vi "Func-엑셀 데이터를 그래프로 출력.vi"() -> ()   [LabVIEW 2015] (continued)
3.3\t3.3\t13.424\n3.3\t3.3\t13.421\n3.3\t3.3\t13.421\n3.3\t3.3\t13.424\n3.3\t3.3\t13.424\n3.3\t3.3\t13.418\n3.3\t3.3\t13.417\n3.3\t3.3\t13.415\n3.3\t3.3\t13.412\n3.3\t3.3\t13.407\n3.3\t3.3\t13.404\n3.3\t3.3\t13.403\n3.3\t3.3\t13.401\n3.3\t3.3\t13.399\n3.3\t3.3\t13.397\n3.3\t3.3\t13.395\n3.3\t3.3\t13.394\n3.3\t3.3\t13.395\n3.3\t3.3\t13.394\n3.3\t3.3\t13.395\n3.3\t3.3\t13.391\n3.3\t3.3\t13.389\n3.3\t3.3\t13.387\n3.3\t3.3\t13.384\n3.3\t3.3\t13.385\n3.3\t3.3\t13.382\n3.3\t3.3\t13.381\n3.3\t3.3\t13.379\n3.3\t3.3\t13.379\n3.3\t3.3\t13.379\n3.3\t3.3\t13.376\n3.3\t3.3\t13.374\n3.3\t3.3\t13.375\n3.3\t3.3\t13.378\n3.3\t3.3\t13.375\n3.3\t3.3\t13.371\n3.3\t3.3\t13.367\n3.3\t3.3\t13.366\n3.3\t3.3\t13.359\n3.3\t3.3\t13.358\n3.3\t3.3\t13.359\n3.3\t3.3\t13.357\n3.3\t3.3\t13.358\n3.3\t3.3\t13.356\n3.3\t3.3\t13.356\n3.3\t3.3\t13.352\n3.3\t3.3\t13.348\n3.3\t3.3\t13.343\n3.3\t3.3\t13.341\n3.3\t3.3\t13.34\n3.3\t3.3\t13.339\n3.3\t3.3\t13.336\n3.3\t3.3\t13.338\n3.3\t3.3\t13.337\n3.3\t3.3\t13.336\n3.3\t3.3\t13.335\n3.3\t3.3\t13.334\n3.3\t3.3\t13.335\n3.3\t3.3\t13.336\n3.3\t3.3\t13.334\n3.3\t3.3\t13.332\n3.3\t3.3\t13.331\n3.3\t3.3\t13.329\n3.3\t3.3\t13.327\n3.3\t3.3\t13.322\n3.3\t3.3\t13.321\n3.3\t3.3\t13.319\n3.3\t3.3\t13.317\n3.3\t3.3\t13.312\n3.3\t3.3\t13.309\n3.3\t3.3\t13.305\n3.3\t3.3\t13.302\n3.3\t3.3\t13.305\n3.3\t3.3\t13.308\n3.3\t3.3\t13.309\n3.3\t3.3\t13.31\n3.3\t3.3\t13.309\n3.3\t3.3\t13.304\n3.3\t3.3\t13.302\n3.3\t3.3\t13.299\n3.3\t3.3\t13.294\n3.3\t3.3\t13.29\n3.3\t3.3\t13.29\n3.3\t3.3\t13.289\n3.3\t3.3\t13.286\n3.3\t3.3\t13.284\n3.3\t3.3\t13.282\n3.3\t3.3\t13.282\n3.3\t3.3\t13.28\n3.3\t3.3\t13.276\n3.3\t3.3\t13.277\n3.3\t3.3\t13.277\n3.3\t3.3\t13.274\n3.3\t3.3\t13.273\n3.3\t3.3\t13.273\n3.3\t3.3\t13.277\n3.3\t3.3\t13.272\n3.3\t3.3\t13.268\n3.3\t3.3\t13.271\n3.3\t3.3\t13.269\n3.3\t3.3\t13.265\n3.3\t3.3\t13.258\n3.3\t3.3\t13.258\n3.3\t3.3\t13.257\n3.3\t3.3\t13.251\n3.3\t3.3\t13.249\n3.3\t3.3\t13.249\n3.3\t3.3\t13.25\n3.3\t3.3\t13.25\n3.3\t3.3\t13.246\n3.3\t3.3\t13.246\n3.3\t3.3\t13.241\n3.3\t3.3\t13.241\n3.3\t3.3\t13.24\n3.3\t3.3\t13.236\n3.3\t3.3\t13.234\n3.3\t3.3\t13.23\n3.3\t3.3\t13.232\n3.3\t3.3\t13.229\n3.3\t3.28\t13.225\n3.3\t3.28\t13.226\n3.3\t3.28\t13.227\n3.3\t3.28\t13.228\n3.3\t3.28\t13.229\n3.3\t3.28\t13.227\n3.3\t3.28\t13.229\n3.3\t3.28\t13.226\n3.3\t3.28\t13.222\n3.3\t3.28\t13.218\n3.3\t3.28\t13.214\n3.3\t3.28\t13.213\n3.3\t3.28\t13.211\n3.3\t3.28\t13.209\n3.3\t3.28\t13.212\n3.3\t3.28\t13.211\n3.3\t3.28\t13.21\n3.3\t3.28\t13.209\n3.3\t3.28\t13.209\n3.3\t3.28\t13.205\n3.3\t3.28\t13.202\n3.3\t3.28\t13.199\n3.3\t3.28\t13.199\n3.3\t3.28\t13.196\n3.3\t3.28\t13.194\n3.3\t3.28\t13.199\n3.3\t3.28\t13.2\n3.3\t3.28\t13.2\n3.3\t3.28\t13.193\n3.3\t3.28\t13.188\n3.3\t3.28\t13.185\n3.3\t3.28\t13.181\n3.3\t3.28\t13.18\n3.3\t3.28\t13.179\n3.3\t3.28\t13.181\n3.3\t3.28\t13.181\n3.3\t3.28\t13.181\n3.3\t3.28\t13.179\n3.3\t3.28\t13.178\n3.3\t3.28\t13.176\n3.3\t3.28\t13.179\n3.3\t3.28\t13.179\n3.3\t3.28\t13.176\n3.3\t3.28\t13.176\n3.3\t3.28\t13.171\n3.3\t3.28\t13.171\n3.3\t3.28\t13.167\n3.3\t3.28\t13.167\n3.3\t3.28\t13.166\n3.3\t3.28\t13.163\n3.3\t3.28\t13.165\n3.3\t3.28\t13.161\n3.3\t3.28\t13.16\n3.3\t3.28\t13.161\n3.3\t3.28\t13.16\n3.3\t3.3\t13.161\n3.3\t3.3\t13.157\n3.3\t3.3\t13.155\n3.3\t3.3\t13.154\n3.3\t3.3\t13.151\n3.3\t3.3\t13.151\n3.3\t3.3\t13.149\n3.3\t3.3\t13.15\n3.3\t3.3\t13.148\n3.3\t3.3\t13.148\n3.3\t3.3\t13.148\n3.3\t3.3\t13.145\n3.3\t3.3\t13.144\n3.3\t3.3\t13.143\n3.3\t3.3\t13.138\n3.3\t3.3\t13.135\n3.3\t3.3\t13.13\n3.3\t3.3\t13.128\n3.3\t3.3\t13.126\n3.3\t3.3\t13.124\n3.3\t3.3\t13.126\n3.3\t3.3\t13.128\n3.3\t3.3\t13.127\n3.3\t3.3\t13.125\n3.3\t3.3\t13.126\n3.3\t3.3\t13.126\n3.3\t3.3\t13.124\n3.3\t3.3\t13.121\n3.3\t3.3\t13.122\n3.3\t3.3\t13.119\n3.3\t3.3\t13.118\n3.3\t3.3\t13.114\n3.3\t3.3\t13.113\n3.3\t3.3\t13.111\n3.3\t3.3\t13.11\n3.3\t3.3\t13.108\n3.3\t3.3\t13.103\n3.3\t3.3\t13.101\n3.3\t3.3\t13.101\n3.3\t3.3\t13.097\n3.3\t3.3\t13.091\n3.3\t3.3\t13.091\n3.3\t3.3\t13.092\n3.3\t3.3\t13.094\n3.3\t3.3\t13.092\n3.3\t3.3\t13.09\n3.3\t3.3\t13.093\n3.3\t3.3\t13.091\n3.3\t3.3\t13.088\n3.3\t3.3\t13.083\n3.3\t3.3\t13.082\n3.3\t3.3\t13.082\n3.3\t3.3\t13.076\n3.3\t3.3\t13.076\n3.3\t3.3\t13.075\n3.3\t3.3\t13.077\n3.3\t3.3\t13.079\n3.3\t3.3\t13.079\n3.3\t3.3\t13.083\n3.3\t3.3\t13.082\n3.3\t3.3\t13.082\n3.3\t3.3\t13.082\n3.3\t3.3\t13.076\n3.3\t3.3\t13.075\n3.3\t3.3\t13.072\n3.3\t3.3\t13.07\n3.3\t3.3\t13.068\n3.3\t3.3\t13.062\n3.3\t3.3\t13.061\n3.3\t3.3\t13.06\n3.3\t3.3\t13.061\n3.3\t3.3\t13.061\n3.3\t3.3\t13.065\n3.3\t3.3\t13.066\n3.3\t3.3\t13.068\n3.3\t3.3\t13.064\n3.3\t3.3\t13.059\n3.3\t3.3\t13.057\n3.3\t3.3\t13.053\n3.3\t3.3\t13.051\n3.3\t3.3\t13.046\n3.3\t3.3\t13.05\n3.3\t3.3\t13.052\n3.3\t3.3\t13.05\n3.3\t3.3\t13.047\n3.3\t3.3\t13.044\n3.3\t3.3\t13.046\n3.3\t3.3\t13.046\n3.3\t3.3\t13.041\n3.3\t3.3\t13.04\n3.3\t3.3\t13.042\n3.3\t3.3\t13.044\n3.3\t3.3\t13.043\n3.3\t3.3\t13.039\n3.3\t3.3\t13.037\n3.3\t3.3\t13.037\n3.3\t3.3\t13.033\n3.3\t3.3\t13.031\n3.3\t3.3\t13.03\n3.3\t3.3\t13.029\n3.3\t3.3\t13.027\n3.3\t3.3\t13.025\n3.3\t3.3\t13.024\n3.3\t3.3\t13.021\n3.3\t3.3\t13.021\n3.3\t3.3\t13.021\n3.3\t3.3\t13.02\n3.3\t3.3\t13.019\n3.3\t3.3\t13.017\n3.3\t3.3\t13.013\n3.3\t3.3\t13.009\n3.3\t3.3\t13.005\n3.3\t3.3\t13.005\n3.3\t3.3\t13.004\n3.3\t3.3\t13.004\n3.3\t3.3\t13.004\n3.3\t3.3\t13.004\n3.3\t3.3\t13.002\n3.3\t3.3\t12.996\n3.3\t3.3\t12.999\n3.3\t3.3\t12.998\n3.3\t3.3\t13\n3.3\t3.3\t12.996\n3.3\t3.3\t12.996\n3.3\t3.3\t13\n3.3\t3.3\t12.998\n3.3\t3.3\t12.997\n3.3\t3.3\t12.995\n3.3\t3.3\t12.995\n3.3\t3.3\t12.995\n3.3\t3.3\t12.99\n3.3\t3.3\t12.985\n3.3\t3.3\t12.985\n3.3\t3.3\t12.982\n3.3\t3.3\t12.98\n3.3\t3.3\t12.981\n3.3\t3.3\t12.986\n3.3\t3.3\t12.989\n3.3\t3.3\t12.988\n3.3\t3.3\t12.987\n3.3\t3.3\t12.989\n3.3\t3.3\t12.985\n3.3\t3.3\t12.977\n3.3\t3.3\t12.976\n3.3\t3.3\t12.972\n3.3\t3.3\t12.971\n3.3\t3.3\t12.971\n3.3\t3.3\t12.972\n3.3\t3.3\t12.971\n3.3\t3.3\t12.968\n3.3\t3.3\t12.968\n3.3\t3.3\t12.966\n3.3\t3.3\t12.964\n3.3\t3.3\t12.963\n3.3\t3.3\t12.961\n3.3\t3.3\t12.962\n3.3\t3.3\t12.964\n3.3\t3.3\t12.964\n3.3\t3.3\t12.962\n3.3\t3.3\t12.961\n3.3\t3.3\t12.961\n3.3\t3.3\t12.961\n3.3\t3.3\t12.959\n3.3\t3.3\t12.956\n3.3\t3.3\t12.954\n3.3\t3.3\t12.952\n3.3\t3.3\t12.954\n3.3\t3.3\t12.951\n3.3\t3.3\t12.95\n3.3\t3.3\t12.951\n3.3\t3.3\t12.948\n3.3\t3.3\t12.948\n3.3\t3.3\t12.943\n3.3\t3.3\t12.941\n3.3\t3.3\t12.941\n3.3\t3.3\t12.938\n3.3\t3.3\t12.94\n3.3\t3.3\t12.941\n3.3\t3.3\t12.941\n3.3\t3.3\t12.939\n3.3\t3.3\t12.934\n3.3\t3.3\t12.934\n3.3\t3.3\t12.93\n3.3\t3.3\t12.929\n3.3\t3.3\t12.925\n3.3\t3.3\t12.924\n3.3\t3.3\t12.929\n3.3\t3.3\t12.927\n3.3\t3.3\t12.929\n3.3\t3.3\t12.923\n3.3\t3.3\t12.92\n3.3\t3.3\t12.922\n3.3\t3.3\t12.92\n3.3\t3.3\t12.919\n3.3\t3.3\t12.919\n3.3\t3.3\t12.922\n3.3\t3.3\t12.925\n3.3\t3.3\t12.924\n3.3\t3.3\t12.923\n3.3\t3.3\t12.918\n3.3\t3.3\t12.916\n3.3\t3.3\t12.914\n3.3\t3.3\t12.906\n3.3\t3.3\t12.904\n3.3\t3.3\t12.902\n3.3\t3.3\t12.902\n3.3\t3.3\t12.903\n3.3\t3.3\t12.902\n3.3\t3.3\t12.904\n3.3\t3.3\t12.901\n3.3\t3.3\t12.9\n3.3\t3.3\t12.899\n3.3\t3.3\t12.898\n3.3\t3.3\t12.898\n3.3\t3.3\t12.901\n3.3\t3.3\t12.899\n3.3\t3.3\t12.896\n3.3\t3.3\t12.898\n3.3\t3.3\t12.895\n3.3\t3.3\t12.893\n3.3\t3.3\t12.889\n3.3\t3.3\t12.891\n3.3\t3.3\t12.89\n3.3\t3.3\t12.885\n3.3\t3.3\t12.884\n3.3\t3.3\t12.885\n3.3\t3.3\t12.882\n3.3\t3.3\t12.88\n3.3\t3.3\t12.88\n3.3\t3.3\t12.878\n3.3\t3.3\t12.878\n3.3\t3.3\t12.878\n3.3\t3.3\t12.879\n3.3\t3.3\t12.878\n3.3\t3.3\t12.877\n3.3\t3.3\t12.879\n3.3\t3.3\t12.875\n3.3\t3.3\t12.873\n3.3\t3.3\t12.871\n3.3\t3.3\t12.871\n3.3\t3.3\t12.871\n3.3\t3.3\t12.871\n3.3\t3.3\t12.87\n3.3\t3.3\t12.863\n3.3\t3.3\t12.864\n3.3\t3.3\t12.862\n3.3\t3.3\t12.863\n3.3\t3.3\t12.862\n3.3\t3.3\t12.862\n3.3\t3.3\t12.865\n3.3\t3.3\t12.862\n3.3\t3.3\t12.864\n3.3\t3.3\t12.862\n3.3\t3.3\t12.859\n3.3\t3.3\t12.857\n3.3\t3.3\t12.857\n3.3\t3.3\t12.859\n3.3\t3.3\t12.854\n3.3\t3.3\t12.855\n3.3\t3.3\t12.854\n3.3\t3.3\t12.854\n3.3\t3.3\t12.854\n3.3\t3.3\t12.853\n3.3\t3.3\t12.853\n3.3\t3.3\t12.846\n3.3\t3.3\t12.849\n3.3\t3.3\t12.846\n3.3\t3.3\t12.843\n3.3\t3.3\t12.836\n3.3\t3.3\t12.835\n3.3\t3.3\t12.837\n3.3\t3.3\t12.833\n3.3\t3.3\t12.83\n3.3\t3.3\t12.83\n3.3\t3.3\t12.833\n3.3\t3.3\t12.831\n3.3\t3.3\t12.826\n3.3\t3.3\t12.826\n3.3\t3.3\t12.828\n3.3\t3.3\t12.826\n3.3\t3.3\t12.826\n3.3\t3.3\t12.827\n3.3\t3.3\t12.831\n3.3\t3.3\t12.83\n3.3\t3.3\t12.826\n3.3\t3.3\t12.827\n3.3\t3.3\t12.825\n3.3\t3.3\t12.823\n3.3\t3.3\t12.822\n3.3\t3.3\t12.821\n3.3\t3.3\t12.823\n3.3\t3.3\t12.821\n3.3\t3.3\t12.819\n3.3\t3.3\t12.82\n3.3\t3.3\t12.815\n3.3\t3.3\t12.814\n3.3\t3.3\t12.816\n3.3\t3.3\t12.815\n3.3\t3.3\t12.816\n3.3\t3.3\t12.812\n3.3\t3.3\t12.816\n3.3\t3.3\t12.815\n3.3\t3.3\t12.811\n3.3\t3.3\t12.811\n3.3\t3.3\t12.812\n3.3\t3.3\t12.817\n3.3\t3.3\t12.811\n3.3\t3.3\t12.809\n3.3\t3.3\t12.808\n3.3\t3.3\t12.805\n3.3\t3.3\t12.8\n3.3\t3.3\t12.799\n3.3\t3.3\t12.8\n3.3\t3.3\t12.803\n3.3\t3.3\t12.805\n3.3\t3.3\t12.805\n3.3\t3.3\t12.807\n3.3\t3.3\t12.805\n3.3\t3.3\t12.802\n3.3\t3.3\t12.796\n3.3\t3.3\t12.79\n3.3\t3.3\t12.79\n3.3\t3.3\t12.791\n3.3\t3.3\t12.788\n3.3\t3.3\t12.791\n3.3\t3.3\t12.793\n3.3\t3.3\t12.795\n3.3\t3.3\t12.795\n3.3\t3.3\t12.793\n3.3\t3.3\t12.796\n3.3\t3.3\t12.791\n3.3\t3.3\t12.792\n3.3\t3.3\t12.789\n3.3\t3.3\t12.791\n3.3\t3.3\t12.789\n3.3\t3.3\t12.787\n3.3\t3.3\t12.786\n3.3\t3.3\t12.784\n3.3\t3.3\t12.783\n3.3\t3.3\t12.779\n3.3\t3.3\t12.777\n3.3\t3.3\t12.779\n3.3\t3.3\t12.78\n3.3\t3.3\t12.779\n3.3\t3.3\t12.778\n3.3\t3.3\t12.781\n3.3\t3.3\t12.783\n3.3\t3.3\t12.778\n3.3\t3.3\t12.776\n3.3\t3.3\t12.776\n3.3\t3.3\t12.776\n3.3\t3.3\t12.77\n3.3\t3.3\t12.767\n3.3\t3.3\t12.766\n3.3\t3.3\t12.769\n3.3\t3.3\t12.768\n3.3\t3.3\t12.765\n3.3\t3.3\t12.766\n3.3\t3.3\t12.763\n3.3\t3.3\t12.762\n3.3\t3.3\t12.759\n3.3\t3.3\t12.761\n3.3\t3.3\t12.761\n3.3\t3.3\t12.757\n3.3\t3.3\t12.758\n3.3\t3.3\t12.76\n3.3\t3.3\t12.762\n3.3\t3.3\t12.759\n3.3\t3.3\t12.76\n3.3\t3.3\t12.761\n3.3\t3.3\t12.761\n3.3\t3.3\t12.759\n3.3\t3.3\t12.752\n3.3\t3.3\t12.748\n3.3\t3.3\t12.749\n3.3\t3.3\t12.746\n3.3\t3.3\t12.743\n3.3\t3.3\t12.744\n3.3\t3.3\t12.748\n3.3\t3.3\t12.746\n3.3\t3.3\t12.744\n3.3\t3.3\t12.743\n3.3\t3.3\t12.744\n3.3\t3.3\t12.741\n3.3\t3.3\t12.736\n3.3\t3.3\t12.737\n3.3\t3.3\t12.738\n3.3\t3.3\t12.738\n3.3\t3.3\t12.735\n3.3\t3.3\t12.738\n3.3\t3.3\t12.737\n3.3\t3.3\t12.733\n3.3\t3.3\t12.73\n3.3\t3.3\t12.73\n3.3\t3.3\t12.729\n3.3\t3.3\t12.727\n3.3\t3.3\t12.727\n3.3\t3.3\t12.727\n3.3\t3.3\t12.73\n3.3\t3.3\t12.73\n3.3\t3.3\t12.731\n3.3\t3.3\t12.729\n3.3\t3.3\t12.727\n3.3\t3.3\t12.727\n3.3\t3.3\t12.72\n3.3\t3.3\t12.72\n3.3\t3.3\t12.716\n3.3\t3.3\t12.714\n3.3\t3.3\t12.717\n3.3\t3.3\t12.717\n3.3\t3.3\t12.72\n3.3\t3.3\t12.718\n3.3\t3.3\t12.718\n3.3\t3.3\t12.721\n3.3\t3.3\t12.716\n3.3\t3.3\t12.718\n3.3\t3.3\t12.714\n3.3\t3.3\t12.716\n3.3\t3.3\t12.715\n3.3\t3.3\t12.713\n3.3\t3.3\t12.715\n3.3\t3.3\t12.709\n3.3\t3.3\t12.709\n3.3\t3.3\t12.706\n3.3\t3.3\t12.705\n3.3\t3.3\t12.704\n3.3\t3.3\t12.698\n3.3\t3.3\t12.703\n3.3\t3.3\t12.702\n3.3\t3.3\t12.701\n3.3\t3.3\t12.702\n3.3\t3.3\t12.704\n3.3\t3.3\t12.706\n3.3\t3.3\t12.704\n3.3\t3.3\t12.705\n3.3\t3.3\t12.705\n3.3\t3.3\t12.704\n3.3\t3.3\t12.701\n3.3\t3.3\t12.7\n3.3\t3.3\t12.699\n3.3\t3.3\t12.696\n3.3\t3.3\t12.697\n3.3\t3.3\t12.697\n3.3\t3.3\t12.695\n3.3\t3.3\t12.693\n3.3\t3.3\t12.692\n3.3\t3.3\t12.694\n3.3\t3.3\t12.693\n3.3\t3.3\t12.695\n3.3\t3.3\t12.697\n3.3\t3.3\t12.694\n3.3\t3.3\t12.692\n3.3\t3.3\t12.69\n3.3\t3.3\t12.689\n3.3\t3.3\t12.681\n3.3\t3.3\t12.677\n3.3\t3.3\t12.677\n3.3\t3.3\t12.676\n3.3\t3.3\t12.673\n3.3\t3.3\t12.673\n3.3\t3.3\t12.677\n3.3\t3.3\t12.682\n3.3\t3.3\t12.68\n3.3\t3.3\t12.678\n3.3\t3.3\t12.677\n3.3\t3.3\t12.67\n3.3\t3.3\t12.669\n3.3\t3.3\t12.661\n3.3\t3.3\t12.66\n3.3\t3.3\t12.661\n3.3\t3.3\t12.659\n3.3\t3.3\t12.664\n3.3\t3.3\t12.663\n3.3\t3.3\t12.662\n3.3\t3.3\t12.661\n3.3\t3.3\t12.658\n3.3\t3.3\t12.659\n3.3\t3.3\t12.655\n3.3\t3.3\t12.654\n3.3\t3.3\t12.654\n3.3\t3.3\t12.653\n3.3\t3.3\t12.656\n3.3\t3.3\t12.659\n3.3\t3.3\t12.657\n3.3\t3.3\t12.659\n3.3\t3.3\t12.659\n3.3\t3.3\t12.663\n3.3\t3.3\t12.659\n3.3\t3.3\t12.656\n3.3\t3.3\t12.656\n3.3\t3.3\t12.654\n3.3\t3.3\t12.652\n3.3\t3.3\t12.651\n3.3\t3.3\t12.653\n3.3\t3.3\t12.65\n3.3\t3.3\t12.651\n3.3\t3.3\t12.656\n3.3\t3.3\t12.656\n3.3\t3.3\t12.651\n3.3\t3.3\t12.652\n3.3\t3.3\t12.652\n3.3\t3.3\t12.65\n3.3\t3.3\t12.645\n3.3\t3.3\t12.645\n3.3\t3.3\t12.648\n3.3\t3.3\t12.646\n3.3\t3.3\t12.647\n3.3\t3.3\t12.646\n3.3\t3.3\t12.643\n3.3\t3.3\t12.641\n3.3\t3.3\t12.639\n3.3\t3.3\t12.636\n3.3\t3.3\t12.636\n3.3\t3.3\t12.639\n3.3\t3.3\t12.643\n3.3\t3.3\t12.643\n3.3\t3.3\t12.644\n3.3\t3.3\t12.643\n3.3\t3.3\t12.641\n3.3\t3.3\t12.64\n3.3\t3.3\t12.633\n3.3\t3.3\t12.632\n3.3\t3.3\t12.632\n3.3\t3.3\t12.632\n3.3\t3.3\t12.633\n3.3\t3.3\t12.632\n3.3\t3.3\t12.635\n3.3\t3.3\t12.634\n3.3\t3.3\t12.631\n3.3\t3.3\t12.629\n3.3\t3.3\t12.628\n3.3\t3.3\t12.625\n3.3\t3.3\t12.625\n3.3\t3.3\t12.625\n3.3\t3.3\t12.628\n3.3\t3.3\t12.628\n3.3\t3.3\t12.628\n3.3\t3.3\t12.629\n3.3\t3.3\t12.63\n3.3\t3.3\t12.63\n3.3\t3.3\t12.628\n3.3\t3.3\t12.626\n3.3\t3.3\t12.624\n3.3\t3.3\t12.625\n3.3\t3.3\t12.622\n3.3\t3.3\t12.621\n3.3\t3.3\t12.616\n3.3\t3.3\t12.613\n3.3\t3.3\t12.613\n3.3\t3.3\t12.609\n3.3\t3.3\t12.608\n3.3\t3.3\t12.608\n3.3\t3.3\t12.611\n3.3\t3.3\t12.615\n3.3\t3.3\t12.612\n3.3\t3.3\t12.611\n3.3\t3.3\t12.614\n3.3\t3.3\t12.613\n3.3\t3.3\t12.612\n3.3\t3.3\t12.61\n3.3\t3.3\t12.609\n3.3\t3.3\t12.609\n3.3\t3.3\t12.607\n3.3\t3.3\t12.611\n3.3\t3.3\t12.61\n3.3\t3.3\t12.61\n3.3\t3.3\t12.612\n3.3\t3.3\t12.61\n3.3\t3.3\t12.611\n3.3\t3.3\t12.607\n3.3\t3.3\t12.606\n3.3\t3.3\t12.603\n3.3\t3.3\t12.601\n3.3\t3.3\t12.6\n3.3\t3.3\t12.598\n3.3\t3.3\t12.601\n3.3\t3.3\t12.601\n3.3\t3.3\t12.6\n3.3\t3.3\t12.604\n3.3\t3.3\t12.602\n3.3\t3.3\t12.6\n3.3\t3.3\t12.593\n3.3\t3.3\t12.593\n3.3\t3.3\t12.588\n3.3\t3.3\t12.586\n3.3\t3.3\t12.585\n3.3\t3.3\t12.585\n3.3\t3.3\t12.584\n3.3\t3.3\t12.584\n3.3\t3.3\t12.587\n3.3\t3.3\t12.585\n3.3\t3.3\t12.587\n3.3\t3.3\t12.589\n3.3\t3.3\t12.587\n3.3\t3.3\t12.583\n3.3\t3.3\t12.585\n3.3\t3.3\t12.583\n3.3\t3.3\t12.584\n3.3\t3.3\t12.579\n3.3\t3.3\t12.583\n3.3\t3.3\t12.59\n3.3\t3.3\t12.589\n3.3\t3.3\t12.588\n3.3\t3.3\t12.582\n3.3\t3.3\t12.584\n3.3\t3.3\t12.585\n3.3\t3.3\t12.58\n3.3\t3.3\t12.58\n3.3\t3.3\t12.582\n3.3\t3.3\t12.585\n3.3\t3.3\t12.583\n3.3\t3.3\t12.577\n3.3\t3.3\t12.574\n3.3\t3.3\t12.573\n3.3\t3.3\t12.567\n3.3\t3.3\t12.567\n3.3\t3.3\t12.57\n3.3\t3.3\t12.571\n3.3\t3.3\t12.573\n3.3\t3.3\t12.575\n3.3\t3.3\t12.576\n3.3\t3.3\t12.577\n3.3\t3.3\t12.575\n3.3\t3.3\t12.575\n3.3\t3.3\t12.571\n3.3\t3.3\t12.568\n3.3\t3.3\t12.567\n3.3\t3.3\t12.568\n3.3\t3.3\t12.567\n3.3\t3.3\t12.567\n3.3\t3.3\t12.568\n3.3\t3.3\t12.567\n3.3\t3.3\t12.569\n3.3\t3.3\t12.566\n3.3\t3.3\t12.567\n3.3\t3.3\t12.566\n3.3\t3.3\t12.566\n3.3\t3.3\t12.565\n3.3\t3.3\t12.563\n3.3\t3.3\t12.562\n3.3\t3.3\t12.557\n3.3\t3.3\t12.553\n3.3\t3.3\t12.551\n3.3\t3.3\t12.552\n3.3\t3.3\t12.55\n3.3\t3.3\t12.55\n3.3\t3.3\t12.554\n3.3\t3.3\t12.556\n3.3\t3.3\t12.554\n3.3\t3.3\t12.55\n3.3\t3.3\t12.548\n3.3\t3.3\t12.548\n3.3\t3.3\t12.546\n3.3\t3.3\t12.545\n3.3\t3.3\t12.547\n3.3\t3.3\t12.55\n3.3\t3.3\t12.554\n3.3\t3.3\t12.551\n3.3\t3.3\t12.552\n3.3\t3.3\t12.549\n3.3\t3.3\t12.547\n3.3\t3.3\t12.548\n3.3\t3.3\t12.541\n3.3\t3.3\t12.545\n3.3\t3.3\t12.542\n3.3\t3.3\t12.545\n3.3\t3.3\t12.543\n3.3\t3.3\t12.542\n3.3\t3.3\t12.545\n3.3\t3.3\t12.544\n3.3\t3.3\t12.541\n3.3\t3.3\t12.538\n3.3\t3.3\t12.542\n3.3\t3.3\t12.541\n3.3\t3.3\t12.539\n3.3\t3.3\t12.538\n3.3\t3.3\t12.539\n3.3\t3.3\t12.54\n3.3\t3.3\t12.537\n3.3\t3.3\t12.537\n3.3\t3.3\t12.535\n3.3\t3.3\t12.532\n3.3\t3.3\t12.529\n3.3\t3.3\t12.53\n3.3\t3.3\t12.53\n3.3\t3.3\t12.527\n3.3\t3.3\t12.526\n3.3\t3.3\t12.529\n3.3\t3.3\t12.528\n3.3\t3.3\t12.528\n3.3\t3.3\t12.527\n3.3\t3.3\t12.529\n3.3\t3.3\t12.526\n3.3\t3.3\t12.525\n3.3\t3.3\t12.528\n3.3\t3.3\t12.525\n3.3\t3.3\t12.521\n3.3\t3.3\t12.522\n3.3\t3.3\t12.525\n3.3\t3.3\t12.527\n3.3\t3.3\t12.523\n3.3\t3.3\t12.525\n3.3\t3.3\t12.527\n3.3\t3.3\t12.526\n3.3\t3.3\t12.526\n3.3\t3.3\t12.526\n3.3\t3.3\t12.527\n3.3\t3.3\t12.526\n3.3\t3.3\t12.524\n3.3\t3.3\t12.523\n3.3\t3.3\t12.523\n3.3\t3.3\t12.523\n3.3\t3.3\t12.521\n3.3\t3.3\t12.523\n3.3\t3.3\t12.524\n3.3\t3.3\t12.526\n3.3\t3.3\t12.523\n3.3\t3.3\t12.517\n3.3\t3.3\t12.517\n3.3\t3.3\t12.512\n3.3\t3.3\t12.513\n3.3\t3.3\t12.511\n3.3\t3.3\t12.514\n3.3\t3.3\t12.517\n3.3\t3.3\t12.516\n3.3\t3.3\t12.521\n3.3\t3.3\t12.517\n3.3\t3.3\t12.516\n3.3\t3.3\t12.513\n3.3\t3.3\t12.516\n3.3\t3.3\t12.518\n3.3\t3.3\t12.516\n3.3\t3.3\t12.514\n3.3\t3.3\t12.512\n3.3\t3.3\t12.513\n3.3\t3.3\t12.508\n3.3\t3.3\t12.503\n3.3\t3.3\t12.5\n3.3\t3.3\t12.498\n3.3\t3.3\t12.5\n3.3\t3.3\t12.5\n3.3\t3.3\t12.503\n3.3\t3.3\t12.504\n3.3\t3.3\t12.503\n3.3\t3.3\t12.504\n3.3\t3.3\t12.503\n3.3\t3.3\t12.503\n3.3\t3.3\t12.504\n3.3\t3.3\t12.504\n3.3\t3.3\t12.504\n3.3\t3.3\t12.504\n3.3\t3.3\t12.505\n3.3\t3.3\t12.504\n3.3\t3.3\t12.499\n3.3\t3.3\t12.501\n3.3\t3.3\t12.502\n3.3\t3.3\t12.502\n3.3\t3.3\t12.5\n3.3\t3.3\t12.502\n3.3\t3.3\t12.503\n3.3\t3.3\t12.498\n3.3\t3.3\t12.494\n3.3\t3.3\t12.496\n3.3\t3.3\t12.491\n3.3\t3.3\t12.489\n3.3\t3.3\t12.49\n3.3\t3.3\t12.493\n3.3\t3.3\t12.491\n3.3\t3.3\t12.491\n3.3\t3.3\t12.493\n3.3\t3.3\t12.49\n3.3\t3.3\t12.488\n3.3\t3.3\t12.486\n3.3\t3.3\t12.487\n3.3\t3.3\t12.484\n3.3\t3.3\t12.483\n3.3\t3.3\t12.479\n3.3\t3.3\t12.477\n3.3\t3.3\t12.478\n3.3\t3.3\t12.477\n3.3\t3.3\t12.478\n3.3\t3.3\t12.479\n3.3\t3.3\t12.48\n3.3\t3.3\t12.48\n3.3\t3.3\t12.48\n3.3\t3.3\t12.487\n3.3\t3.3\t12.488\n3.3\t3.3\t12.488\n3.3\t3.3\t12.491\n3.3\t3.3\t12.493\n3.3\t3.3\t12.493\n3.3\t3.3\t12.486\n3.3\t3.3\t12.483\n3.3\t3.3\t12.48\n3.3\t3.3\t12.479\n3.3\t3.3\t12.477\n3.3\t3.3\t12.476\n3.3\t3.3\t12.478\n3.3\t3.3\t12.478\n3.3\t3.3\t12.477\n3.3\t3.3\t12.477\n3.3\t3.3\t12.475\n3.3\t3.3\t12.474\n3.3\t3.3\t12.473\n3.3\t3.3\t12.47\n3.3\t3.3\t12.473\n3.3\t3.3\t12.473\n3.3\t3.3\t12.476\n3.3\t3.3\t12.478\n3.3\t3.3\t12.475\n3.3\t3.3\t12.477\n3.3\t3.3\t12.474\n3.3\t3.3\t12.473\n3.3\t3.3\t12.469\n3.3\t3.3\t12.465\n3.3\t3.3\t12.468\n3.3\t3.3\t12.468\n3.3\t3.3\t12.468\n3.3\t3.3\t12.469\n3.3\t3.3\t12.468\n3.3\t3.3\t12.471\n3.3\t3.3\t12.466\n3.3\t3.3\t12.464\n3.3\t3.3\t12.46\n3.3\t3.3\t12.461\n3.3\t3.3\t12.461\n3.3\t3.3\t12.46\n3.3\t3.3\t12.462\n3.3\t3.3\t12.463\n3.3\t3.3\t12.463\n3.3\t3.3\t12.46\n3.3\t3.3\t12.464\n3.3\t3.3\t12.461\n3.3\t3.3\t12.462\n3.3\t3.3\t12.464\n3.3\t3.3\t12.466\n3.3\t3.3\t12.469\n3.3\t3.3\t12.467\n3.3\t3.3\t12.467\n3.3\t3.3\t12.465\n3.3\t3.3\t12.465\n3.3\t3.3\t12.464\n3.3\t3.3\t12.462\n3.3\t3.3\t12.464\n3.3\t3.3\t12.465\n3.3\t3.3\t12.466\n3.3\t3.3\t12.46\n3.3\t3.3\t12.461\n3.3\t3.3\t12.461\n3.3\t3.3\t12.457\n3.3\t3.3\t12.454\n3.3\t3.3\t12.451\n3.3\t3.3\t12.454\n3.3\t3.3\t12.45\n3.3\t3.3\t12.448\n3.3\t3.3\t12.448\n3.3\t3.3\t12.452\n3.3\t3.3\t12.454\n3.3\t3.3\t12.45\n3.3\t3.3\t12.452\n3.3\t3.3\t12.451\n3.3\t3.3\t12.449\n3.3\t3.3\t12.448\n3.3\t3.3\t12.446\n3.3\t3.3\t12.448\n3.3\t3.3\t12.45\n3.3\t3.3\t12.452\n3.3\t3.3\t12.451\n3.3\t3.3\t12.45\n3.3\t3.3\t12.45\n3.3\t3.3\t12.451\n3.3\t3.3\t12.447\n3.3\t3.3\t12.447\n3.3\t3.3\t12.444\n3.3\t3.3\t12.443\n3.3\t3.3\t12.443\n3.3\t3.3\t12.438\n3.3\t3.3\t12.439\n3.3\t3.3\t12.437\n3.3\t3.3\t12.439\n3.3\t3.3\t12.441\n3.3\t3.3\t12.443\n3.3\t3.3\t12.446\n3.3\t3.3\t12.447\n3.3\t3.3\t12.447\n3.3\t3.3\t12.445\n3.3\t3.3\t12.446\n3.3\t3.3\t12.442\n3.3\t3.3\t12.437\n3.3\t3.3\t12.435\n3.3\t3.3\t12.432\n3.3\t3.3\t12.433\n3.3\t3.3\t12.432\n3.3\t3.3\t12.43\n3.3\t3.3\t12.432\n3.3\t3.3\t12.437\n3.3\t3.3\t12.44\n3.3\t3.3\t12.437\n3.3\t3.3\t12.435\n3.3\t3.3\t12.436\n3.3\t3.3\t12.439\n3.3\t3.3\t12.433\n3.3\t3.3\t12.431\n3.3\t3.3\t12.435\n3.3\t3.3\t12.434\n3.3\t3.3\t12.433\n3.3\t3.3\t12.434\n3.3\t3.3\t12.437\n3.3\t3.3\t12.439\n3.3\t3.3\t12.436\n3.3\t3.3\t12.437\n3.3\t3.3\t12.436\n3.3\t3.3\t12.434\n3.3\t3.3\t12.429\n3.3\t3.3\t12.429\n3.3\t3.3\t12.43\n3.3\t3.3\t12.43\n3.3\t3.3\t12.43\n3.3\t3.3\t12.429\n3.3\t3.3\t12.432\n3.3\t3.3\t12.431\n3.3\t3.3\t12.43\n3.3\t3.3\t12.43\n3.3\t3.3\t12.43\n3.3\t3.3\t12.429\n3.3\t3.3\t12.425\n3.3\t3.3\t12.427\n3.3\t3.3\t12.425\n3.3\t3.3\t12.423\n3.3\t3.3\t12.422\n3.3\t3.3\t12.425\n3.3\t3.3\t12.425\n3.3\t3.3\t12.422\n3.3\t3.3\t12.422\n3.3\t3.3\t12.424\n3.3\t3.3\t12.421\n3.3\t3.3\t12.415\n3.3\t3.3\t12.418\n3.3\t3.3\t12.418\n3.3\t3.3\t12.417\n3.3\t3.3\t12.418\n3.3\t3.3\t
